vi "Broadcast Diagnostic.vi"(9 "CAN Offset":u32=512 format="%x", 11 "CANTXQueueIn":T1) -> (3 "CANTXQueueOut":T1)   [LabVIEW 2015]
uses:
  TX Library/CAN Message Queue.ctl
  TX Library/CAN Message.ctl
  TX Library/Transmit CAN.vi
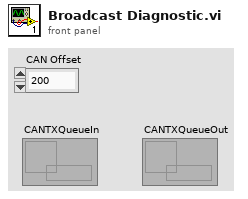
[diagram p1: front panel]
types:
  T1 = typedef "CAN Message Queue.ctl" = refnum<k33>
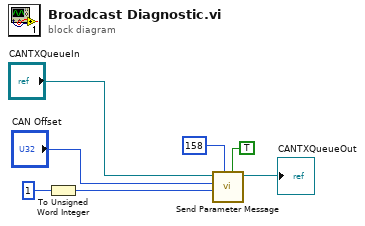
[diagram p0: block diagram]
diagram:
  n1 = To Unsigned Word Integer(number=u16 1) -> (unsigned 16bit integer=w4:u16)
  n2 = call "Send Parameter Message.vi"("Write?"=TRUE, "Param Address"=i16 158, "Data"=w4, "CAN Offset"="CAN Offset", "CANTXQueueIn"="CANTXQueueIn") -> ("CANTXQueueOut"=→"CANTXQueueOut":T1)  [unwired: 6 in]
